vi "Работа с CVS( exel) файлом knob.vi"() -> ()   [LabVIEW 2021]
uses:
  <vilib>/Utility/file.llb/Write Delimited Spreadsheet (DBL).vi
  <vilib>/Utility/file.llb/Read Delimited Spreadsheet (DBL).vi
panel:
  out "all rows":dbl[][](array[numeric])
  in  "file path (dialog if empty)":path
  in  "Knob":dbl(knob) scale=0.0..10.0
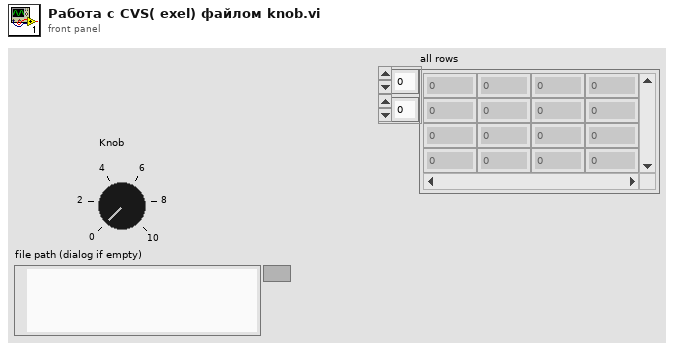
[diagram p1: front panel]
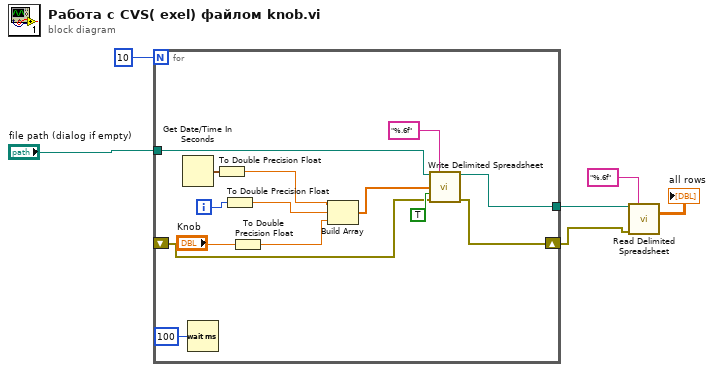
[diagram p0: block diagram]
diagram:
  n1 = for {
    N: 10 -> [_]
    shift-right: [w11] -> w3
    shift-left: _ -> [w9]
    tunnel: "file path (dialog if empty)" -> [w10]
    tunnel: [w7] -> w4
    i -> [w15]
    n2 = Get Date/Time In Seconds() -> (seconds since 1Jan1904=w19:timestamp)
    n3 = Wait (ms)(milliseconds to wait=u32 100) -> ()  [unwired: 1 out]
    n4 = To Double Precision Float(number=w19) -> (double precision float=w18:dbl)
    n5 = To Double Precision Float(number=w15) -> (double precision float=w17:dbl)
    n6 = To Double Precision Float(number="Knob") -> (double precision float=w16:dbl)
    n7 = Build Array(w18, w17, w16) -> (w8:dbl[])
    n8 = call-poly <vilib>:"Write Delimited Spreadsheet.vi"("file path (dialog if empty)"=w10, "format (%.3f)"="%.6f", "1D data"=w8, "append to file? (new file:F)"=TRUE, "error in (no error)"=w9) -> ("new file path (Not A Path if cancelled)"=w7:path, "error out"=w11:errorcluster)  [unwired: 9 in]
  }
  n9 = call-poly <vilib>:"Read Delimited Spreadsheet.vi"("file path (dialog if empty)"=w4, "format (%.3f)"="%.6f", "error in (no error)"=w3) -> ("all rows"=→"all rows":dbl[][])  [unwired: 7 in, 5 out]
